vi "Write Sensor Index.vi"(8 "error in (no error)":errorcluster, 10 "Sensor Index":i32, 11 "Realsense Cam in":refnum<class "Realsense Cam.lvclass">) -> (0 "error out":errorcluster, 3 "Realsense Cam out":refnum<class "Realsense Cam.lvclass">)   [LabVIEW 2018, in "Realsense Cam.lvclass"]
uses:
  Realsense Cam.lvclass
  Realsense Cam.lvclass/Realsense Cam.ctl
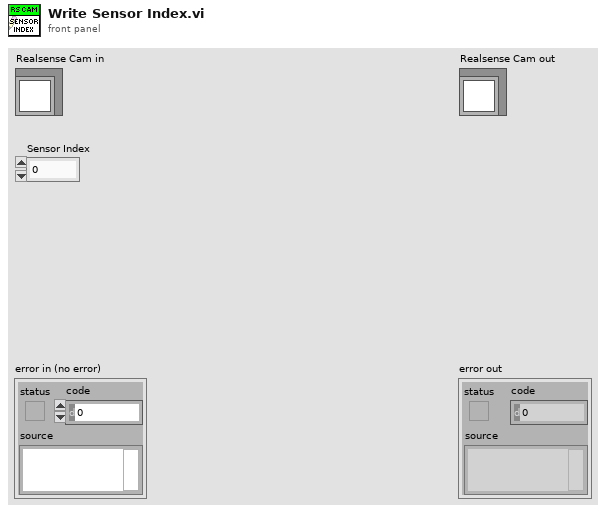
[diagram p1: front panel]
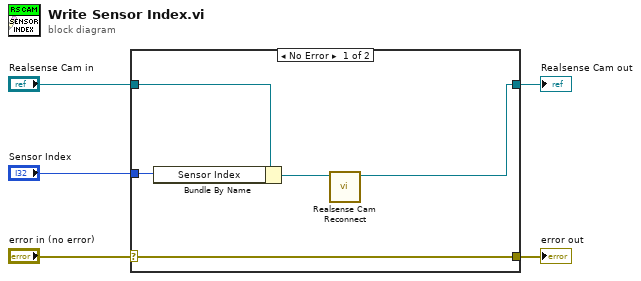
[diagram p0: block diagram]
diagram:
  n1 = case shown="No Error" "error in (no error)" {
    selector: "error in (no error)" -> [w10 w11]
    tunnel: [w10 w11] -> w4
    tunnel: [w6 w12] -> w2
    tunnel: "Realsense Cam in" -> [w9 w12]
    tunnel: "Sensor Index" -> [w8 _]
    frame No Error {
      n2 = Bundle By Name(cluster=w9, "Sensor Index"=w8) -> (w7:refnum<class "Realsense Cam.lvclass">)
      n3 = call-dynamic "Realsense Cam Reconnect.vi"("Realsense Cam in"=w7) -> ("Realsense Cam out"=w6:refnum<class "Realsense Cam.lvclass">)  [unwired: 7 in, 3 out]
    }
    frame Error {
    }
  }
  "error out" <- w4
  "Realsense Cam out" <- w2
